vi "SetActiveAuto.vi"(1 "ActiveAutoRoutine":string, 2 "ActiveStartPosition":string) -> ()   [LabVIEW 2017]
uses:
  <vilib>/Rock Robotics/Network Tables/NT Write String.vi
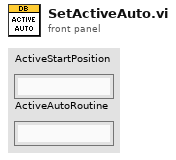
[diagram p1: front panel]
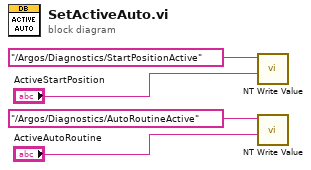
[diagram p0: block diagram]
diagram:
  n1 = call-poly <vilib>:"NT Write Value.vi"("String"="ActiveStartPosition", "Name"="/Argos/Diagnostics/StartPositionActive") -> ()  [unwired: 9 in, 1 out]
  n2 = call-poly <vilib>:"NT Write Value.vi"("String"="ActiveAutoRoutine", "Name"="/Argos/Diagnostics/AutoRoutineActive") -> ()  [unwired: 9 in, 1 out]
